vi "DAQ_PW_Set_check_Vbat.vi"(6 "Vbat_set":dbl, 7 "DEV_BUSY":T1, 8 "error in (no error)":errorcluster, 9 "DUT Voltage Selector":enum16{"3.8VDC", "2.9VDC", "By Pass", "4.0VDC"}(ring), 10 "DAQmx Device Name":tag, 11 "OUTPUT":bool) -> (3 "JSON string":string)   [LabVIEW 2015]
uses:
  Share Data/uPower_kit.ctl
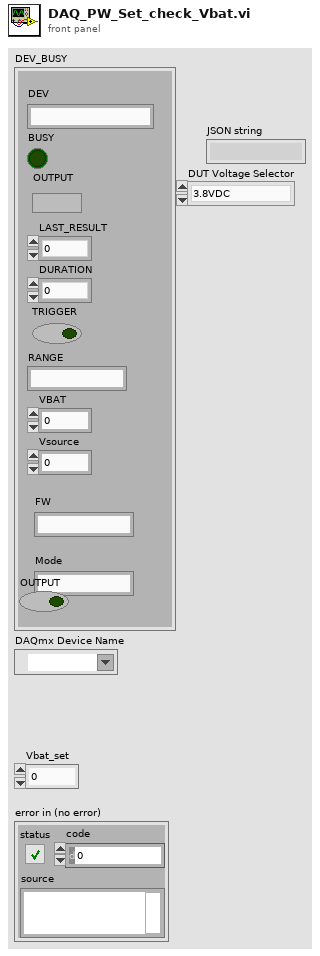
[diagram p1: front panel]
types:
  T1 = typedef "uPower_kit.ctl" = cluster{"DEV":string, "BUSY":bool, "VBAT":dbl, "OUTPUT":bool, "LAST_RESULT":dbl, "DURATION":u16, "TRIGGER":bool, "RANGE":string, "Vsource":dbl, "FW":string, "Mode":string}
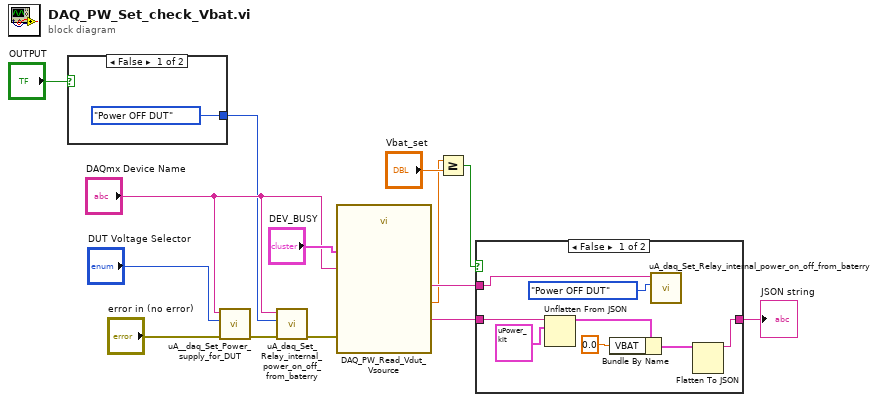
[diagram p0: block diagram]
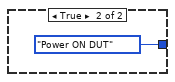
[diagram p3: hidden frame]
diagram:
  n1 = case shown="False" "OUTPUT" {
    tunnel: [enum16{"Power ON DUT", "Power OFF DUT"}."Power OFF DUT" ("Power ON/OFF DUT") enum16{"Power ON DUT", "Power OFF DUT"}."Power ON DUT" ("Power ON/OFF DUT")] -> w3
    frame False {
    }
    frame True {
    }
  }
  n2 = call "uA__daq_Set_Power_supply_for_DUT.vi"("error in"="error in (no error)", "DUT Voltage Selector"="DUT Voltage Selector", "USB DAQ"="DAQmx Device Name") -> ("error out"=w2:errorcluster)  [unwired: 8 in]
  n3 = call "uA_daq_Set_Relay_internal_power_on_off_from_baterry.vi"("error in"=w2, "Power ON/OFF DUT"=w3, "USB DAQ"="DAQmx Device Name") -> ("error out"=w1:errorcluster)  [unwired: 8 in]
  n4 = call "DAQ_PW_Read_Vdut_Vsource.vi"("error in (no error)"=w1, "DEV_BUSY"="DEV_BUSY", "DAQmx Device Name"="DAQmx Device Name") -> ("DAQmx Device Name ou"=w14:tag, "Vsource"=w9:dbl, "JSON string"=w12:string)  [unwired: 6 in]
  n5 = Greater Or Equal?(x=w9, y="Vbat_set") -> (x >= y?=w11:bool)
  n6 = case shown="False" w11 {
    tunnel: w14 -> [w24 _]
    tunnel: w12 -> [w22 w25]
    tunnel: [w17 w25] -> w13
    frame False {
      n7 = Unflatten From JSON(JSON string=w22, type and defaults=T1 {"DEV"="", "BUSY"=FALSE, "VBAT"=0.0, "OUTPUT"=FALSE, "LAST_RESULT"=0.0, "DURATION"=0, "TRIGGER"=FALSE, "RANGE"="", "Vsource"=0.0, "FW"="", "Mode"=""} ("DEV_BUSY 2")) -> (value=w20:T1)  [unwired: 5 in, 1 out]
      n8 = Bundle By Name(cluster=w20, "VBAT"=0.0) -> (w18:T1)
      n9 = call "uA_daq_Set_Relay_internal_power_on_off_from_baterry.vi"("Power ON/OFF DUT"=enum16{"Power ON DUT", "Power OFF DUT"}."Power OFF DUT", "USB DAQ"=w24) -> ()  [unwired: 9 in, 1 out]
      n10 = Flatten To JSON(anything=w18) -> (JSON string=w17:string)  [unwired: 2 in, 1 out]
    }
    frame True {
    }
  }
  "JSON string" <- w13
